vi "System Initialize.vi"(10 "UI References":T1) -> (0 "error out":errorcluster, 2 "UI Console Out":refnum<class "UI Console.lvclass">)   [LabVIEW 2019]
uses:
  TypeDef/Messenger Factory Type.ctl
  TypeDef/System Factory Type.ctl
  Ancestor Class/Messenger Factory/Messenger Factory.lvclass
  Ancestor Class/System Modules Factory/System Modules Factory.lvclass
  Ancestor Class/Actor/System Actor/System Actor.lvclass
  General Parent Class/UI Console/UI Console.lvclass
  Ancestor Class/Actor/Root Actor/Root Actor.lvclass
  C:/Users/iio/Desktop/NTHU Brain Center/General Purpose/Classes/Ancestor/Actor/System Actor/System Actor.lvclass
  C:/Users/iio/Desktop/NTHU Brain Center/General Purpose/Classes/Ancestor/Actor/Root Actor/Root Actor.lvclass
  TypeDef/UI References.ctl
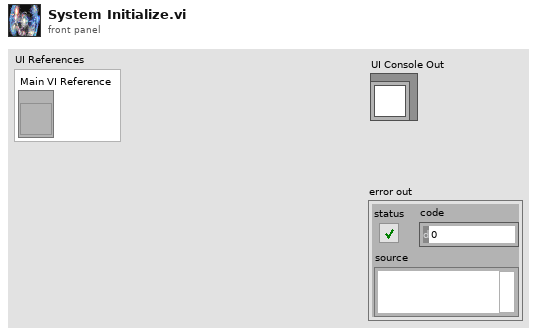
[diagram p1: front panel]
types:
  T1 = typedef "UI References.ctl" = cluster{"Main VI Reference":refnum<vi>}
  T2 = typedef "System Factory Type.ctl" = enum16{"None"}
  T3 = typedef "Messenger Factory Type.ctl" = enum16{"None"}
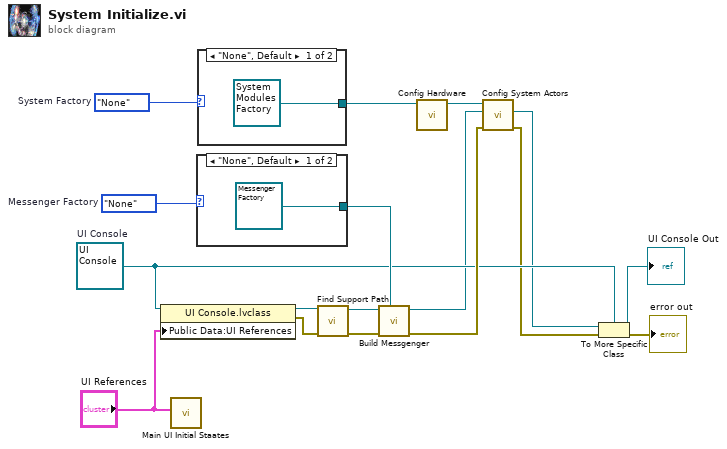
[diagram p0: block diagram]
diagram:
  w6 = refnum<class "UI Console.lvclass"> refnum  # UI Console
  w16 = System_Factory_Type."None"  # System Factory
  w17 = Messenger_Factory_Type."None"  # Messenger Factory
  n1 = property class="UI Console.lvclass"(reference=w6, "Public Data:UI References"="UI References") -> (reference out=w15:refnum<class "UI Console.lvclass">, error out=w14:errorcluster)  [unwired: 1 in]
  n2 = call "Main UI Initial Staates.vi"("UI References"="UI References") -> ()  [unwired: 11 in]
  n3 = case shown="\"None\", Default" w17 {
    tunnel: [refnum<class "Messenger Factory.lvclass"> refnum ("Messenger Factory.lvclass") _] -> w10
    frame "None", Default {
    }
    frame "None" {
    }
  }
  n4 = case shown="\"None\", Default" w16 {
    tunnel: [refnum<class "System Modules Factory.lvclass"> refnum ("System Modules Factory.lvclass") _] -> w9
    frame "None", Default {
    }
    frame "None" {
    }
  }
  n5 = call "Find Support Path.vi"("error in (no error)"=w14, "System Actor in"=w15) -> ("error out"=w12:errorcluster, "System Actor out"=w11:refnum<class "UI Console.lvclass">)  [unwired: 8 in]
  n6 = call-dynamic "Build Messgenger.vi"("Messenger Factory in"=w10, "error in (no error)"=w12, "Root Actor In"=w11) -> ("error out"=w7:errorcluster, "Root Actor Out"=w2:refnum<class "Root Actor.lvclass">)  [unwired: 6 in, 1 out]
  n7 = call-dynamic "Config Hardware.vi"("System Modules Factory in"=w9) -> ("System Modules Factory out"=w8:refnum<class "System Modules Factory.lvclass">)  [unwired: 9 in, 1 out]
  n8 = call-dynamic "Config System Actors.vi"("error in (no error)"=w7, "Root Actor In"=w2, "System Modules Factory in"=w8) -> ("error out"=w5:errorcluster, "Root Actor Out"=w1:refnum<class "Root Actor.lvclass">)  [unwired: 6 in, 1 out]
  n9 = To More Specific Class(target class=w6, reference=w1, error in=w5) -> (specific class reference=→"UI Console Out":refnum<class "UI Console.lvclass">, error out=→"error out":errorcluster)
